vi "Run App.vi"(8 "error in (no error)":errorcluster, 11 "VolatusCore in":refnum<class "VolatusCore.lvclass">) -> (0 "error out":errorcluster, 3 "VolatusCore out":refnum<class "VolatusCore.lvclass">)   [LabVIEW 2020, in "Volatus.lvlib" / "VolatusCore.lvclass"]
uses:
  VolatusCore.lvclass
  VolatusCore.lvclass/VolatusCore.ctl
  App/App.lvclass
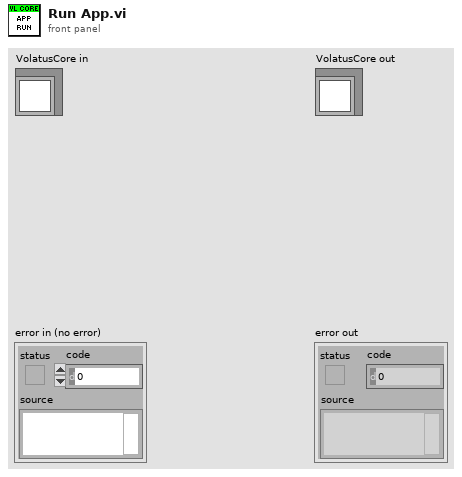
[diagram p1: front panel]
types:
  T1 = typedef "Volatus.lvlib/VolatusCore.lvclass/Startup Notification.ctl" = cluster{"Start":bool, "App":refnum<class "App.lvclass">, "Core APIs":T2}
  T2 = typedef "Volatus.lvlib/Core APIs.ctl" = cluster{"Volatus":refnum<class "VolatusAPI.lvclass">, "Event":refnum<class "EventAPI.lvclass">, "Config":refnum<class "ConfigAPI.lvclass">}
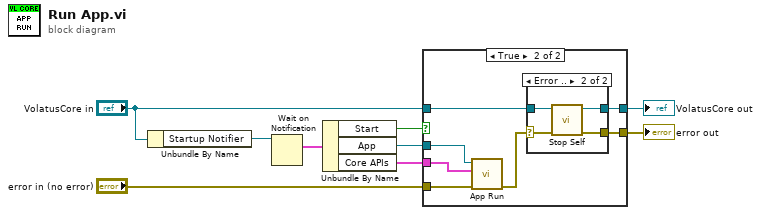
[diagram p0: block diagram]
diagram:
  n1 = Unbundle By Name("VolatusCore in") -> ("Startup Notifier"=w5:refnum<notifier>)
  n2 = Wait on Notification(notifier=w5) -> (notification=w4:T1)  [unwired: 3 in, 3 out]
  n3 = Unbundle By Name(w4) -> ("Start"=w3:bool, "App"=w2:refnum<class "App.lvclass">, "Core APIs"=w1:T2)
  n4 = case shown="True" w3 {
    tunnel: "error in (no error)" -> [w10 w18]
    tunnel: "VolatusCore in" -> [w11 w17]
    tunnel: [w11 w16] -> w7
    tunnel: [w10 w14] -> w6
    tunnel: w2 -> [_ w13]
    tunnel: w1 -> [_ w12]
    frame False {
    }
    frame True {
      n5 = call-dynamic "App Run.vi"("error in (no error)"=w18, "Core APIs"=w12, "App in"=w13) -> ("error out"=w15:errorcluster)  [unwired: 8 in]
      n6 = case shown="Error .." w15 {
        selector: w15 -> [w19 w22]
        tunnel: w17 -> [w20 w24]
        tunnel: [w20 w23] -> w16
        tunnel: [w19 w21] -> w14
        frame No Error {
        }
        frame Error {
          n7 = call "Stop Self.vi"("error in (no error)"=w22, "VolatusCore in"=w24) -> ("error out"=w21:errorcluster, "VolatusCore out"=w23:refnum<class "VolatusCore.lvclass">)  [unwired: 8 in]
        }
      }
    }
  }
  "error out" <- w6
  "VolatusCore out" <- w7
